vi "Keithley2100.measure 2w resistance.vi"(0 "i ref in":refnum<vi>, 1 "Custom Range (100mV)":dbl=0.1 min=0.1 max=1000.0 format="%#.6e", 2 "Digital Filter (0: Off)":u16(ring) items=["Off", "Moving Filter", "Repeating Filter"], 3 "Digital Filter Readings (10)":i32=10, 4 "NPLC":u16(ring)=2 items=[".02", ".1", "1", "10"], 5 "error in (no error)":errorcluster, 9 "Auto Range":bool) -> (14 "i refout":refnum<vi>, 16 "Measurement":dbl format="%#_6e", 19 "error out":errorcluster)   [LabVIEW 2014, in "Keithley2100.lvlib"]
doc: "This VI is used to get the USB port of the USBSwitchBox from the database.\n\nLicense Agreement for this software:\n\nCopyright (C)\nGesellschaft für Schwerionenforschung, GSI\nPlanckstr. 1\n64291 Darmstadt\nGermany\n\nContact: D.Beck@gsi.de \n\nThis program is free software; you can redistribute it and/or modify it under the terms of the \nGNU General Public License as published by the Free Software Foundation; either version 2 of \nthe license, or (at your option) any later version.\n\nThis program is distributed in the hope that it will be useful, but WITHOUT ANY WARRANTY; \nwithout even the implied warranty of MERCHANTABILITY or FITNESS FOR A PARTICULAR PURPOSE. See the GNU General License for more details (http://www.gnu.org).\n\nGesellschaft für Schwerionenforschung, GSI\nPlanckstr. 1, 64291 Darmstadt, Germany\nFor all questions and ideas contact: M.Richter@gsi.de, H.Brand@gsi.de or D.Beck@gsi.de.\nLast update: 16-JUN-2004"
uses:
  Keithley2100.lvlib
  instr.lib/Keithley-2100-Series/Keithley 2100 Series.lvlib
  CSlibraries-extern/DimLVEvent/LVDimInterface/LVDimInterface.lvlib
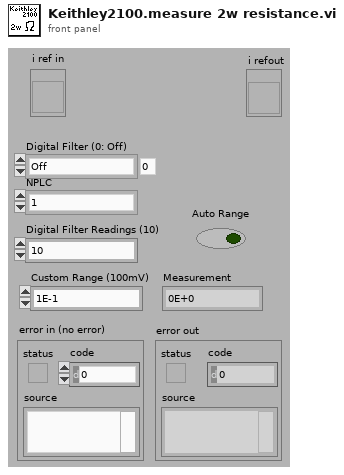
[diagram p1: front panel]
types:
  T1 = typedef "Keithley2100.lvlib/Keithley2100.i attribute.ctl" = cluster{"Custom Range":dbl, "Threshold Range":dbl, "VISA resource name":refnum<visa-resource-name>, "Auto Range":bool, "Digital Filter Readings":i32, "Digital Filter":u16, "NPLC":u16, "Display on":u16, "Resolution":u16, "Beaper enabled":bool, "MeasurementID":i32}
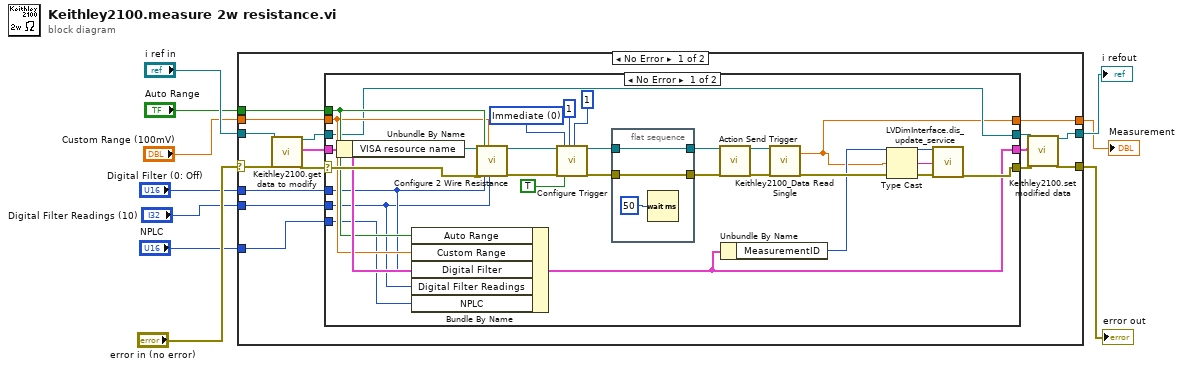
[diagram p0: block diagram]
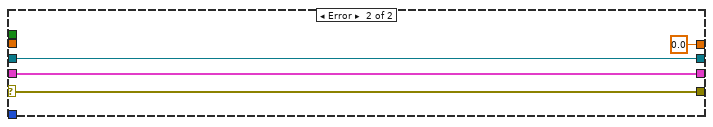
[diagram p2: hidden frame]
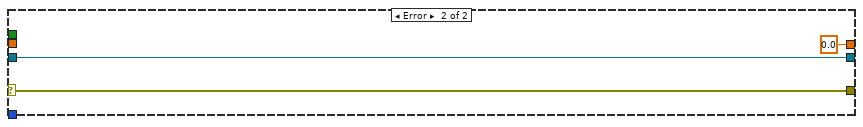
[diagram p3: hidden frame]
diagram:
  n1 = case shown="No Error" "error in (no error)" {
    selector: "error in (no error)" -> [w25 w63]
    tunnel: [w20 w63] -> w8
    tunnel: "i ref in" -> [w26 w62]
    tunnel: [w21 w62] -> w7
    tunnel: "Auto Range" -> [w16 _]
    tunnel: "Custom Range (100mV)" -> [w15 _]
    tunnel: "Digital Filter (0: Off)" -> [w14 _]
    tunnel: "Digital Filter Readings (10)" -> [w13 _]
    tunnel: "NPLC" -> [w12 _]
    tunnel: [w11 0.0 ("Measurement")] -> w1
    frame No Error {
      n2 = call "Keithley2100.get data to modify.vi"("i ref in"=w26, "error in (no error)"=w25) -> ("i ref out"=w23:refnum<vi>, "i attribute"=w22:T1, "error out"=w24:errorcluster)  [unwired: 14 in, 1 out]
      n3 = case shown="No Error" w24 {
        selector: w24 -> [w52 w59]
        tunnel: w23 -> [w33 w60]
        tunnel: w22 -> [w51 w58]
        tunnel: [w33 w60] -> w19
        tunnel: [w31 w59] -> w18
        tunnel: [w30 w58] -> w17
        tunnel: w16 -> [w50 _]
        tunnel: w15 -> [w49 _]
        tunnel: w14 -> [w48 _]
        tunnel: w13 -> [w47 _]
        tunnel: w12 -> [w46 _]
        tunnel: [w28 0.0 ("Measurement")] -> w11
        frame No Error {
          w41 = u16 0 items=["Immediate", "Bus", "External"] ("Source (0: Immediate)")
          n4 = Unbundle By Name(w51) -> ("VISA resource name"=w53:refnum<visa-resource-name>)
          n5 = Bundle By Name(cluster=w51, "Auto Range"=w50, "Custom Range"=w49, "Digital Filter"=w48, "Digital Filter Readings"=w47, "NPLC"=w46) -> (w30:T1)
          n6 = call "Configure 2 Wire Resistance.vi"("VISA resource name"=w53, "error in (no error)"=w52, "Auto Range? (T: Auto)"=w50, "Digital Filter (0: Off)"=w48, "Custom Range (100 Ohm)"=w49, "Digital Filter Readings (10)"=w47) -> ("VISA resource name out"=w45:refnum<visa-resource-name>, "error out"=w44:errorcluster)  [unwired: 12 in]
          n7 = call "Configure Trigger.vi"("VISA resource name"=w45, "error in (no error)"=w44, "Source (0: Immediate)"=w41, "Auto Delay? (T: Auto)"=TRUE, "Sample Count (1)"=1, "Trigger Count (1)"=1) -> ("VISA resource name out"=w39:refnum<visa-resource-name>, "error out"=w38:errorcluster)  [unwired: 12 in]
          n8 = flat-sequence {
            tunnel: [w55] -> w37
            tunnel: w39 -> [w55]
            tunnel: [w54] -> w36
            tunnel: w38 -> [w54]
            frame #0 {
              n9 = Wait (ms)(milliseconds to wait=u32 50) -> ()  [unwired: 1 out]
            }
          }
          n10 = call "Action Send Trigger.vi"("VISA resource name"=w37, "error in (no error)"=w36) -> ("VISA resource name out"=w35:refnum<visa-resource-name>, "error out"=w34:errorcluster)  [unwired: 16 in]
          n11 = Unbundle By Name(w30) -> ("MeasurementID"=w29:i32)
          n12 = call "Keithley2100_Data Read Single.vi"("VISA resource name"=w35, "error in (no error)"=w34) -> ("Measurement"=w28:dbl, "error out"=w32:errorcluster)  [unwired: 15 in, 1 out]
          n13 = Type Cast(x=w28) -> (*(type *) &x=w27:string)  [unwired: 1 in]
          n14 = call "LVDimInterface.dis_update_service.vi"("my_serviceID"=w29, "data"=w27, "error in (no error)"=w32) -> ("error out"=w31:errorcluster)  [unwired: 14 in, 2 out]
        }
        frame Error {
        }
      }
      n15 = call "Keithley2100.set modified data.vi"("i ref in"=w19, "i attribute"=w17, "error in (no error)"=w18) -> ("i ref out"=w21:refnum<vi>, "error out"=w20:errorcluster)  [unwired: 15 in]
    }
    frame Error {
    }
  }
  "error out" <- w8
  "i refout" <- w7
  "Measurement" <- w1
